vi "Launch Sequence Editor.vi"(4 "Environment":path, 5 "Architecture":T1, 6 "wait for reply (T)":bool=TRUE, 7 "Version":string, 8 "error in":errorcluster, 9 "IProcess Executor.lvclass":refnum<class "IProcess Executor.lvclass">, 10 "ITSDiscovery.lvclass":refnum<class "ITSDiscovery.lvclass">) -> (0 "error out":errorcluster, 1 "timed out?":bool)   [LabVIEW 2025, in "TS Environment Manager.lvlib"]
doc: "Launches the Sequence Editor for the specified TS version optionally with the specified environment.\n\n_____\nCreated using DQMH Framework: Event Scripter 7.1.1.1528."
uses:
  TS Environment Manager.lvlib
  ITSDiscovery/ITSDiscovery.lvclass
  IProcess Executor/IProcess Executor.lvclass
  Type Definitions/Architecture--enum.ctl
  Launch Sequence Editor Argument--cluster.ctl
  Launch Sequence Editor (Reply Payload)--cluster.ctl
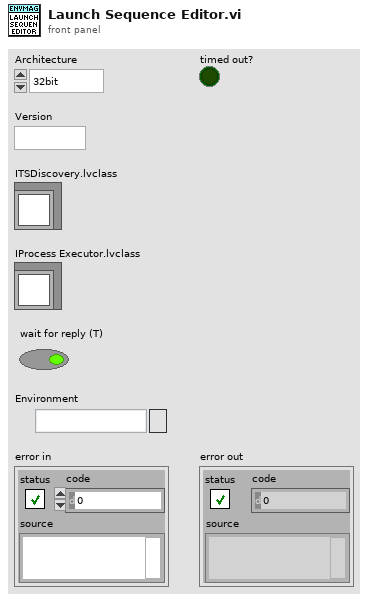
[diagram p1: front panel]
types:
  T1 = typedef "Architecture--enum.ctl" = enum16{"32bit", "64bit"}
  T2 = typedef "TS Environment Manager.lvlib/Launch Sequence Editor Argument--cluster.ctl" = cluster{"ITSDiscovery.lvclass":refnum<class "ITSDiscovery.lvclass">, "IProcess Executor.lvclass":refnum<class "IProcess Executor.lvclass">, "Version":string, "Architecture":T1, "Environment":path, "Wait Notifier":refnum<notifier>, "wait for reply":bool}
  T3 = typedef "TS Environment Manager.lvlib/Request Events--cluster.ctl" = cluster{"Stop Module":refnum<user-event>, "Show Panel":refnum<user-event>, "Hide Panel":refnum<user-event>, "Get Module Execution Status":refnum<user-event>, "Show Diagram":refnum<user-event>, "Get Installations":refnum<user-event>, "Private.Get Profiles File":refnum<user-event>, "Launch Sequence Editor":refnum<user-event>, "Activate Version":refnum<user-event>, "Add Profile":refnum<user-event>, "Get Profile(s)":refnum<user-event>, "Delete Profile":refnum<user-event>, "Set Profiles File":refnum<user-event>}
  T4 = typedef "TS Environment Manager.lvlib/Launch Sequence Editor (Reply Payload)--cluster.ctl" = cluster{"error":errorcluster, "Version":string, "Architecture":T1, "Environment":path}
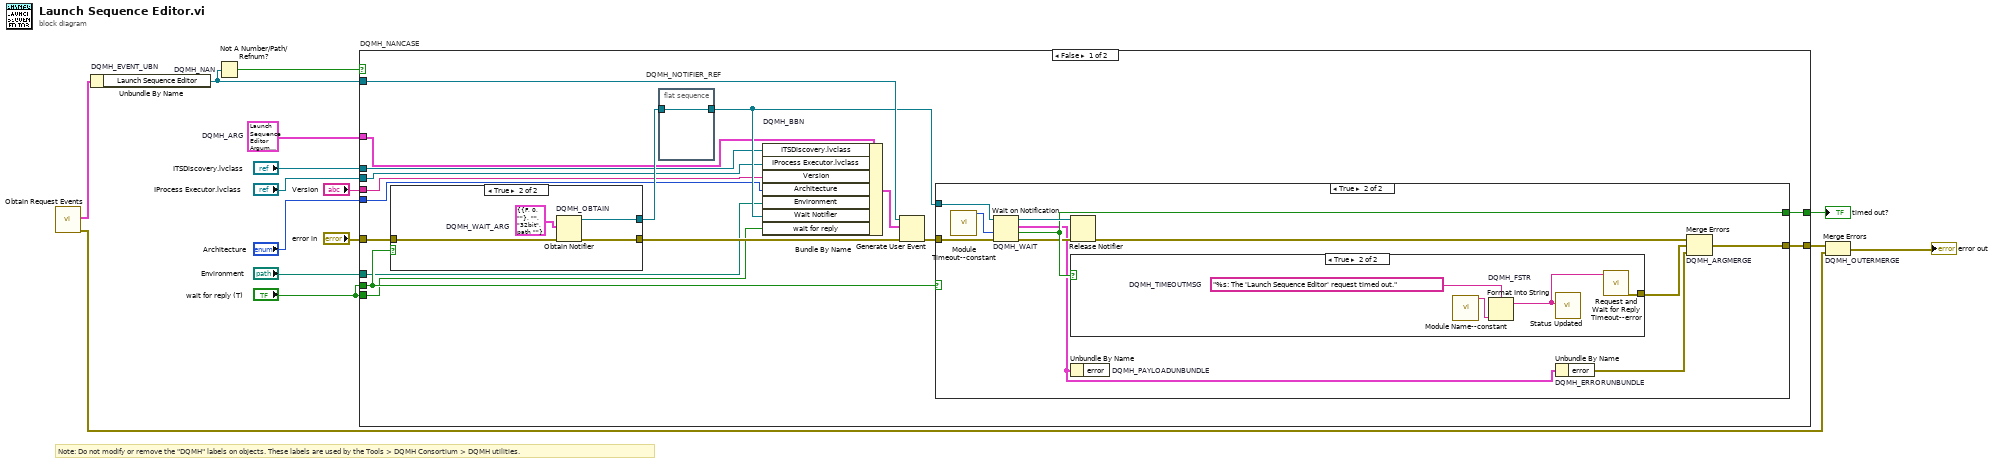
[diagram p0: block diagram]
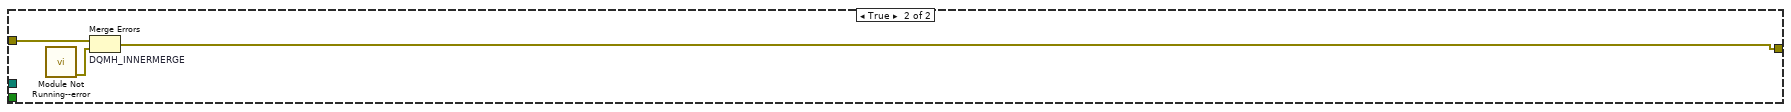
[diagram p5: hidden frame]
diagram:
  w9 = T2 {"ITSDiscovery.lvclass"=refnum, "IProcess Executor.lvclass"=refnum, "Version"="", "Architecture"=enum."32bit", "Environment"=path "", "Wait Notifier"=refnum, "wait for reply"=FALSE}  # DQMH_ARG
  # "Note: Do not modify or remove the \"DQMH\" labels on objects. These labels are used by the Tools > DQMH Consortium > DQMH utilities."
  n1 = call "Obtain Request Events.vi"() -> ("error out"=w2:errorcluster, "TS Environment Manager Request Events"=w1:T3)  [unwired: 10 in]
  n2 = Unbundle By Name "DQMH_EVENT_UBN"(w1) -> ("Launch Sequence Editor"=w10:refnum<user-event>)
  n3 = Not A Number/Path/Refnum? "DQMH_NAN"(number/path/refnum=w10) -> (NaN/Path/Refnum?=w11:bool)
  n4 = case "DQMH_NANCASE" shown="False" w11 {
    tunnel: "error in" -> [w32 w57]
    tunnel: w10 -> [w30 _]
    tunnel: [w27 w56] -> w12
    tunnel: [w28 _] -> w14
    tunnel: "wait for reply (T)" -> [w25 _]
    tunnel: w9 -> [w22 _]
    tunnel: "ITSDiscovery.lvclass" -> [w21 _]
    tunnel: "IProcess Executor.lvclass" -> [w20 _]
    tunnel: "Version" -> [w19 _]
    tunnel: "Architecture" -> [w18 _]
    tunnel: "Environment" -> [w17 _]
    tunnel: "wait for reply (T)" -> [w16 _]
    frame False {
      n5 = case shown="True" w25 {
        tunnel: w32 -> [w50 w54]
        tunnel: [w50 w53] -> w29
        tunnel: [_ w51] -> w24
        frame False {
        }
        frame True {
          w52 = T4 {"error"={"status"=FALSE, "code"=0, "source"=""}, "Version"="", "Architecture"=enum."32bit", "Environment"=path ""}  # DQMH_WAIT_ARG
          n6 = Obtain Notifier "DQMH_OBTAIN"(notification data type=w52, error in (no error)=w54) -> (notifier out=w51:refnum<notifier>, error out=w53:errorcluster)  [unwired: 2 in, 1 out]
        }
      }
      n7 = flat-sequence "DQMH_NOTIFIER_REF" {
        tunnel: w24 -> [w33]
        tunnel: [w33] -> w23
        frame #0 {
        }
      }
      n8 = Bundle By Name "DQMH_BBN"(cluster=w22, "ITSDiscovery.lvclass"=w21, "IProcess Executor.lvclass"=w20, "Version"=w19, "Architecture"=w18, "Environment"=w17, "Wait Notifier"=w23, "wait for reply"=w16) -> (w26:T2)
      n9 = Generate User Event(user event=w30, event data cluster=w26, error in=w29) -> (error out=w31:errorcluster)  [unwired: 1 in, 1 out]
      n10 = case shown="True" w25 {
        tunnel: w31 -> [w34 w45]
        tunnel: w23 -> [_ w44]
        tunnel: [_ w42] -> w28
        tunnel: [w34 w41] -> w27
        frame False {
        }
        frame True {
          n11 = call "Module Timeout--constant.vi"() -> ("Module Timeout"=w35:i32)  [unwired: 11 in]
          n12 = Wait on Notification "DQMH_WAIT"(notifier=w44, timeout in ms (-1)=w35, error in (no error)=w45) -> (notifier out=w43:refnum<notifier>, notification=w36:T4, timed out?=w42:bool, error out=w40:errorcluster)  [unwired: 1 in]
          n13 = Release Notifier(notifier=w43, error in (no error)=w40) -> (error out=w39:errorcluster)  [unwired: 1 in, 2 out]
          n14 = case shown="True" w42 {
            tunnel: [_ w47] -> w37
            frame False {
            }
            frame True {
              w49 = "%s: The 'Launch Sequence Editor' request timed out."  # DQMH_TIMEOUTMSG
              n15 = call "Module Name--constant.vi"() -> ("Module Name"=w46:string)  [unwired: 11 in]
              n16 = Format Into String "DQMH_FSTR"(format string=w49, w46) -> (resulting string=w48:string)  [unwired: 2 in, 1 out]
              n17 = call "Status Updated.vi"("Status"=w48) -> ()  [unwired: 10 in, 1 out]
              n18 = call "Request and Wait for Reply Timeout--error.vi"("Error Message"=w48) -> ("error out"=w47:errorcluster)  [unwired: 10 in]
            }
          }
          n19 = Unbundle By Name "DQMH_PAYLOADUNBUNDLE"(w36) -> ()  [unwired: 1 out]
          n20 = Unbundle By Name "DQMH_ERRORUNBUNDLE"(w36) -> ("error"=w38:errorcluster)
          n21 = Merge Errors "DQMH_ARGMERGE"(w39, w37, w38) -> (w41:errorcluster)
        }
      }
    }
    frame True {
      n22 = call "Module Not Running--error.vi"() -> ("error out"=w55:errorcluster)  [unwired: 11 in]
      n23 = Merge Errors "DQMH_INNERMERGE"(w57, w55) -> (w56:errorcluster)
    }
  }
  "timed out?" <- w14
  n24 = Merge Errors "DQMH_OUTERMERGE"(w12, w2) -> (→"error out":errorcluster)
